vi "shift_point_by_heading.vi"(9 "Distance (m)":dbl, 10 "Heading (deg)":dbl, 11 "UTM Point":T1 {"North" format="%#_10f"; "East" format="%#_8f"}) -> (3 "Shifted UTM Point":T1 {"North" format="%#_10f"; "East" format="%#_8f"})   [LabVIEW 2013]
doc: "This VI takes a heading and distance (deg and m) and shifts the given UTM point by that amount. Ignores hemisphere and zone.\n\nEric Schneider, September 2014"
uses:
  Data/TypeDefs/UTM Location.ctl
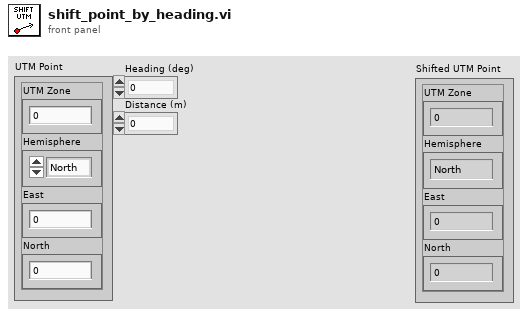
[diagram p1: front panel]
types:
  T1 = typedef "UTM Location.ctl" = cluster{"UTM Zone":dbl, "Hemisphere":enum16{"North", "South"}, "East":dbl, "North":dbl}
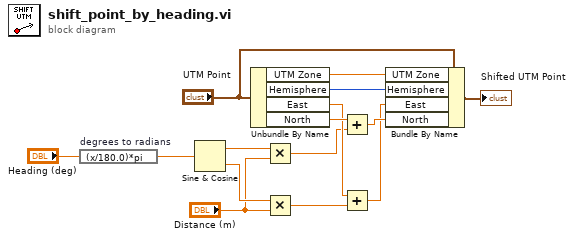
[diagram p0: block diagram]
diagram:
  n1 = expression code="(x/180.0)*pi" "degrees to radians"("Heading (deg)") -> (w14:dbl)
  n2 = Sine & Cosine(0:w14) -> (1:w4:dbl, 2:w6:dbl)
  n3 = Unbundle By Name("UTM Point") -> ("UTM Zone"=w12:dbl, "Hemisphere"=w11:enum16{"North", "South"}, "East"=w8:dbl, "North"=w10:dbl)
  n4 = Multiply(x=w4, y="Distance (m)") -> (x*y=w2:dbl)
  n5 = Multiply(x=w6, y="Distance (m)") -> (x*y=w5:dbl)
  n6 = Add(x=w10, y=w2) -> (x+y=w9:dbl)
  n7 = Add(x=w8, y=w5) -> (x+y=w7:dbl)
  n8 = Bundle By Name(cluster="UTM Point", "UTM Zone"=w12, "Hemisphere"=w11, "East"=w7, "North"=w9) -> (→"Shifted UTM Point":T1)
